vi "Y.vi"(0 "Y":dbl(graph)) -> ()   [LabVIEW 2014]
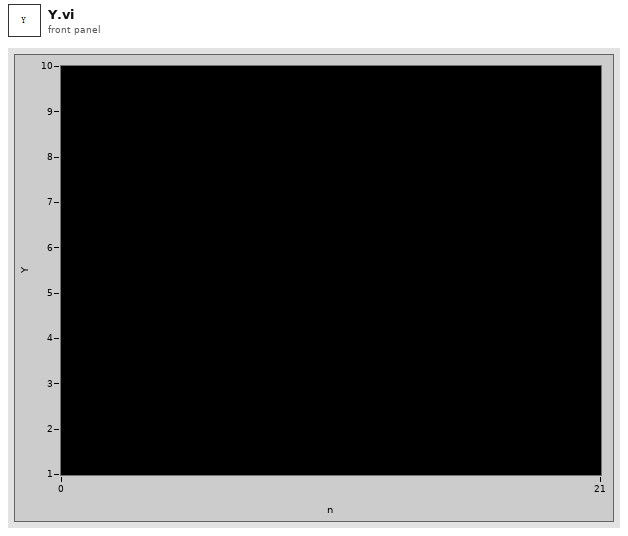
[diagram p1: front panel]
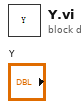
[diagram p0: block diagram]
diagram:
